vi "UpdateFBVarSet.vi"(1 "Variable":T1, 2 "CurrentVarSet":T2) -> (0 "UpdatedVarSet":T2)   [LabVIEW 2013]
uses:
  FBVarSet.ctl
  FBVar.ctl
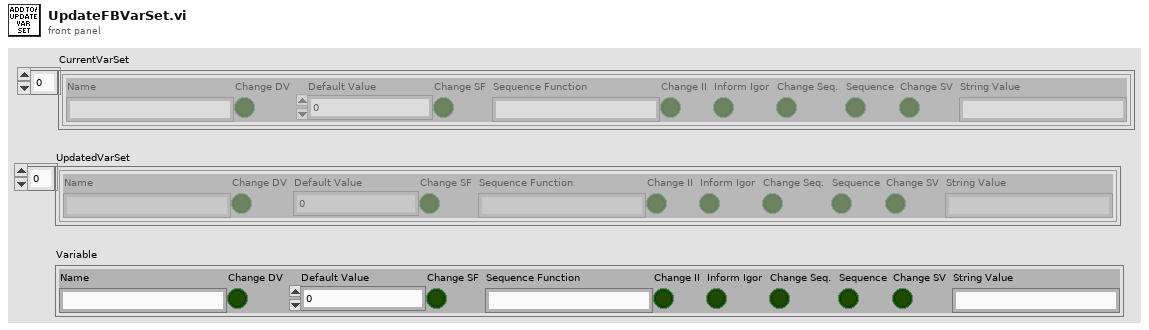
[diagram p1: front panel]
types:
  T1 = typedef "FBVar.ctl" = cluster{"Name":string, "Change DV":bool, "Default Value":dbl, "Change SF":bool, "Sequence Function":string, "Change II":bool, "Inform Igor":bool, "Change Seq.":bool, "Sequence":bool, "Change SV":bool, "String Value":string}
  T2 = typedef "FBVarSet.ctl" = T1[]
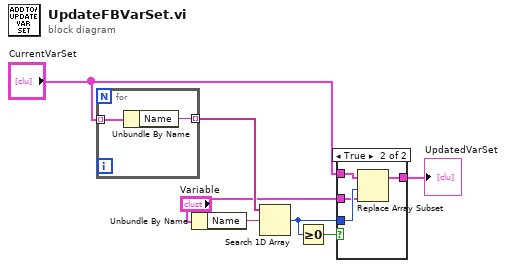
[diagram p0: block diagram]
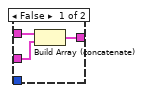
[diagram p2: hidden frame]
diagram:
  n1 = for {
    tunnel: "CurrentVarSet" -> [w9] mode=indexing
    tunnel: [w8] -> w7 mode=indexing
    n2 = Unbundle By Name(w9) -> ("Name"=w8:string)
  }
  n3 = Unbundle By Name("Variable") -> ("Name"=w6:string)
  n4 = Search 1D Array(1D array=w7, element=w6) -> (index of element=w3:i32)  [unwired: 1 in]
  n5 = Greater Or Equal To 0?(x=w3) -> (x >= 0?=w5:bool)
  n6 = case shown="True" w5 {
    tunnel: "CurrentVarSet" -> [w12 w16]
    tunnel: w3 -> [_ w15]
    tunnel: "Variable" -> [w11 w14]
    tunnel: [w10 w13] -> w2
    frame False {
      n7 = Build Array (concatenate)(w12, w11) -> (w10:T2)
    }
    frame True {
      n8 = Replace Array Subset(array=w16, new element=w14, index=w15) -> (w13:T2)
    }
  }
  "UpdatedVarSet" <- w2
